vi "niRFUtil MT UTIL FIR Coefficients.vi"(0 "sampling freq: fs":dbl=1.0 format="%.2f", 1 "filter type":T1(ring), 2 "high cutoff freq: fh":dbl=0.45 format="%.2f", 3 "low cutoff freq: fl":dbl=0.125 format="%.2f", 4 "taps":i32=25) -> (5 "FIR Coefficients":dbl[](array[numeric]) min=0.0 max=127.0 format="%.2f", 6 "error":i32)   [LabVIEW 2015, in "niRFUtil.lvlib"]
doc: "Generates the set of coefficients to implement an FIR filter."
uses:
  niRFUtil.lvlib
  <resource>/lvanlys.dll
panel:
  # "FIR Filter Coefficients"
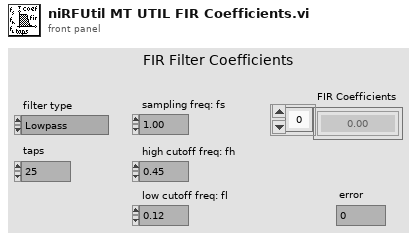
[diagram p1: front panel]
types:
  T1 = enum32{"Lowpass", "Highpass", "Bandpass", "Bandstop"}
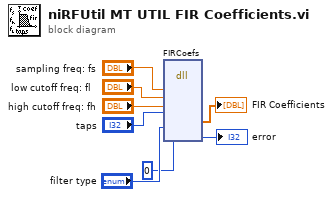
[diagram p0: block diagram]
diagram:
  n1 = dll-call lib="C:/Program Files/National Instruments/LabVIEW 2015/resource/lvanlys.*" fn="FIRCoefs"("fs"="sampling freq: fs", "fl"="low cutoff freq: fl", "fh"="high cutoff freq: fh", "taps"="taps", "type"="filter type", "err"=0) -> ("FIR Coefficients"=→"FIR Coefficients":dbl[], "err"=→"error":i32)  [unwired: 8 in, 4 out]
